vi "Send Instrument String Command.vi"(6 "message attributes":T1, 7 "Comm":refnum<class "VeriStand Comm.lvclass">, 8 "error in (no error)":errorcluster, 10 "Response Parameters":T2, 11 "Command":string) -> (0 "error out":errorcluster)   [LabVIEW 2020, in "Instrument Addon Engine.lvlib"]
uses:
  Instrument Addon Engine.lvlib
  Addon Shared/Types/Response RT Configuration Cluster.ctl
  Addon Shared/Types/Response Parameters.ctl
  Addon Shared/Types/Linked Channel Cluster.ctl
  Addon Shared/Types/Response Wait Type.ctl
  <vilib>/NI/NI VeriStand Addon Network Comm/Engine/VeriStand Comm.lvclass
  <vilib>/NI/Tools/Keyed Array/KeyedArray.ctl
  Addon Shared/Types/Buffered RT Instrument Command.ctl
  <vilib>/NI/NI VeriStand Addon Network Comm/Engine/VeriStand Comm.lvclass/VeriStand Comm.ctl
  <vilib>/NI/AMC/Send Local Message.vi
  Addon Shared/Instrument Addon Shared.lvlib
  <vilib>/NI/Tools/Keyed Array/Tools_KeyedArray.lvlib
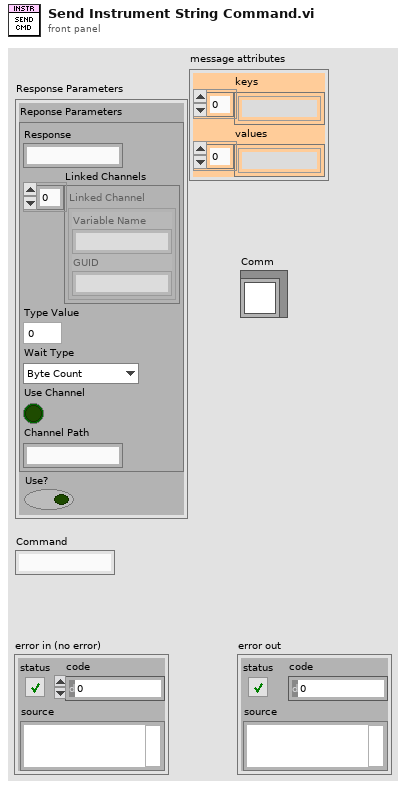
[diagram p1: front panel]
types:
  T1 = typedef "Tools_KeyedArray.lvlib/KeyedArray.ctl" = cluster{"keys":string[], "values":string[]}
  T2 = typedef "Instrument Addon Shared.lvlib/Response RT Configuration Cluster.ctl" = cluster{"Reponse Parameters":T3, "Use?":bool}
  T3 = typedef "Instrument Addon Shared.lvlib/Response Parameters.ctl" = cluster{"Response":string, "Linked Channels":T4[], "Type Value":dbl, "Wait Type":T5, "Use Channel":bool, "Channel Path":string}
  T4 = typedef "Instrument Addon Shared.lvlib/Linked Channel Cluster.ctl" = cluster{"Variable Name":string, "GUID":string}
  T5 = typedef "Instrument Addon Shared.lvlib/Response Wait Type.ctl" = enum16{"Byte Count", "Wait sec"}
  T6 = typedef "Instrument Addon Shared.lvlib/Buffered RT Instrument Command.ctl" = cluster{"Command":string, "Response Expected?":bool, "Wait Type":T5, "Wait Value":dbl}
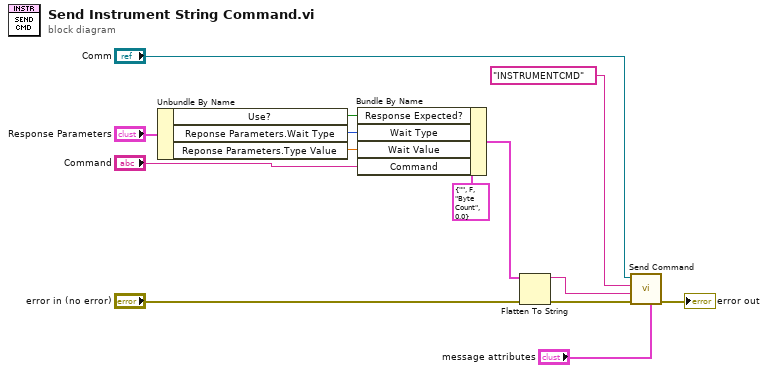
[diagram p0: block diagram]
diagram:
  n1 = Unbundle By Name("Response Parameters") -> ("Use?"=w14:bool, "Reponse Parameters.Wait Type"=w13:T5, "Reponse Parameters.Type Value"=w12:dbl)
  n2 = Bundle By Name(cluster=T6 {"Command"="", "Response Expected?"=FALSE, "Wait Type"=enum."Byte Count", "Wait Value"=0.0}, "Response Expected?"=w14, "Wait Type"=w13, "Wait Value"=w12, "Command"="Command") -> (w10:T6)
  n3 = Flatten To String(anything=w10, error in (no error)="error in (no error)") -> (data string=w8:string, error out=w9:errorcluster)  [unwired: 2 in, 1 out]
  n4 = call <vilib>:"Send Command.vi"("message attributes"="message attributes", "error in (no error)"=w9, "message value"=w8, "message name"="INSTRUMENTCMD", "VeriStand Comm in"="Comm") -> ("error out"=→"error out":errorcluster)  [unwired: 5 in, 1 out]
